vi "Generic command handler.vi"(8 "error in (no error)":errorcluster, 10 "Message in":refnum<class "GenericMessage.lvclass">, 11 "Cascade in":refnum<class "Cascade.lvclass">) -> (0 "error out":errorcluster, 2 "value":string, 3 "Cascade out":refnum<class "Cascade.lvclass">)   [LabVIEW 2012, in "Cascade.lvclass"]
doc: "The generic_command_handler processes the command 'generic'. Commands which are not part of the predefined list of commands fall under the 'generic' command for special activity."
uses:
  Cascade.lvclass
  <vilib>/Distrio/Murmex/GenericMessage/GenericMessage.lvclass
  <vilib>/Distrio/Murmex/Murmex/Murmex.lvclass
  Cascade.lvclass/Cascade.ctl
  <vilib>/Distrio/Murmex/ProceedMessage/ProceedMessage.lvclass
panel:
  # "This method is called when the GENERIC\ntrigger is sent. \n\nOverride this method when your component needs to\nrespond to this trigger. \n\nCall parent for proper implementation"
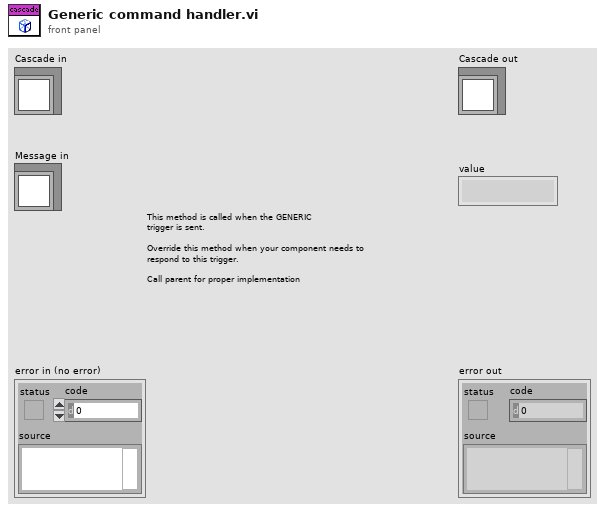
[diagram p1: front panel]
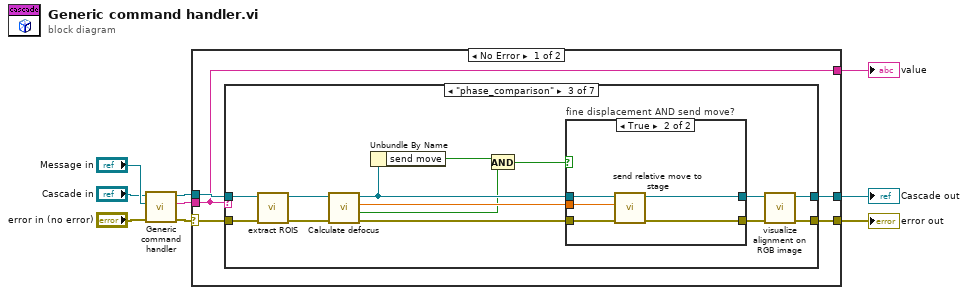
[diagram p0: block diagram]
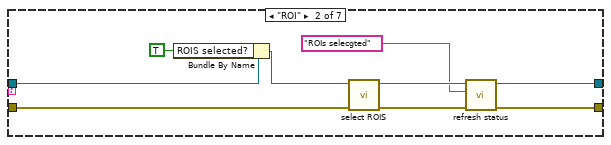
[diagram p3: hidden frame]
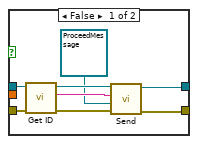
[diagram p4: hidden frame]
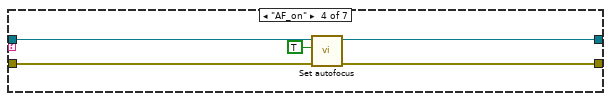
[diagram p5: hidden frame]
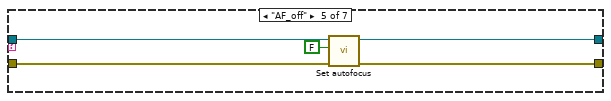
[diagram p6: hidden frame]
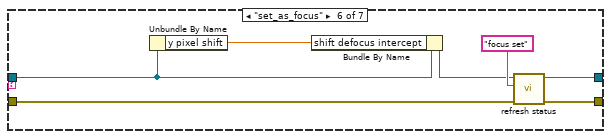
[diagram p7: hidden frame]
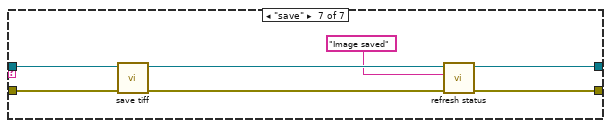
[diagram p8: hidden frame]
diagram:
  n1 = call-parent "Generic command handler.vi"("error in (no error)"="error in (no error)", "Message in"="Message in", "Murmex in"="Cascade in") -> ("error out"=w6:errorcluster, "value"=w4:string, "Murmex out"=w5:refnum<class "Cascade.lvclass">)  [unwired: 6 in]
  n2 = case shown="No Error" w6 {
    selector: w6 -> [w14 w78]
    tunnel: w5 -> [w13 w79]
    tunnel: w4 -> [w12 w77]
    tunnel: [w12 w77] -> w3
    tunnel: [w11 w78] -> w2
    tunnel: [w10 w79] -> w1
    frame No Error {
      n3 = case shown="\"phase_comparison\"" w12 {
        tunnel: w14 -> [w16 w23 w39 w57 w62 w64 w76]
        tunnel: w13 -> [w15 w19 w38 w55 w60 w66 w75]
        tunnel: [w16 w24 w29 w56 w61 w69 w73] -> w11
        tunnel: [w15 w25 w27 w54 w59 w68 w71] -> w10
        frame "False", Default {
        }
        frame "ROI" {
          n4 = Bundle By Name(cluster=w19, "ROIS selected?"=TRUE ("runtime.ROIS selected?")) -> (w18:refnum<class "Cascade.lvclass">)
          n5 = call-dynamic "select ROIS.vi"("error in (no error)"=w23, "Cascade in"=w18) -> ("error out"=w22:errorcluster, "Cascade out"=w21:refnum<class "Cascade.lvclass">)  [unwired: 8 in]
          n6 = call-dynamic "refresh status.vi"("error in (no error)"=w22, "String In"="ROIs selecgted", "Cascade in"=w21) -> ("error out"=w24:errorcluster, "Cascade out"=w25:refnum<class "Cascade.lvclass">)  [unwired: 7 in]
        }
        frame "phase_comparison" {
          n7 = call-dynamic "extract ROIS.vi"("error in (no error)"=w39, "Cascade in"=w38) -> ("error out"=w37:errorcluster, "Cascade out"=w35:refnum<class "Cascade.lvclass">)  [unwired: 8 in]
          n8 = call-dynamic "Calculate defocus.vi"("error in (no error)"=w37, "Cascade in"=w35) -> ("error out"=w36:errorcluster, "fine?"=w30:bool, "translation out"=w33:dbl[unit], "Cascade out"=w34:refnum<class "Cascade.lvclass">)  [unwired: 6 in]
          n9 = Unbundle By Name(w34) -> ("send move"=w32:bool)
          n10 = And(x=w32, y=w30) -> (x .and. y?=w31:bool)
          n11 = case "fine displacement AND send move?" shown="True" w31 {
            tunnel: [w44 w52] -> w28
            tunnel: [w45 w51] -> w26
            tunnel: w34 -> [w46 w50]
            tunnel: w36 -> [w47 w49]
            tunnel: w33 -> [_ w48]
            frame False {
              n12 = call <vilib>:"Get ID.vi"("error in (no error)"=w47, "Murmex in"=w46) -> ("error out"=w43:errorcluster, "component id"=w41:string, "Murmex out"=w42:refnum<class "Cascade.lvclass">)  [unwired: 7 in]
              n13 = call <vilib>:"Send.vi"("error in (no error)"=w43, "Message"=refnum<class "ProceedMessage.lvclass"> refnum ("Distrio Murmex 1.5:ProceedMessage"), "recipient"=w41, "Murmex in"=w42) -> ("error out"=w44:errorcluster, "Murmex out"=w45:refnum<class "Cascade.lvclass">)  [unwired: 6 in]
            }
            frame True {
              n14 = call-dynamic "send relative move to stage.vi"("error in (no error)"=w49, "move to send"=w48, "Cascade in"=w50) -> ("error out"=w52:errorcluster, "Cascade out"=w51:refnum<class "Cascade.lvclass">)  [unwired: 7 in]
            }
          }
          n15 = call-dynamic "visualize alignment on RGB image.vi"("error in (no error)"=w28, "Cascade in"=w26) -> ("error out"=w29:errorcluster, "Cascade out"=w27:refnum<class "Cascade.lvclass">)  [unwired: 8 in]
        }
        frame "AF_on" {
          n16 = call-dynamic "Set autofocus.vi"("error in (no error)"=w57, "autofocusing?"=TRUE, "Cascade in"=w55) -> ("error out"=w56:errorcluster, "Cascade out"=w54:refnum<class "Cascade.lvclass">)  [unwired: 7 in]
        }
        frame "AF_off" {
          n17 = call-dynamic "Set autofocus.vi"("error in (no error)"=w62, "autofocusing?"=FALSE, "Cascade in"=w60) -> ("error out"=w61:errorcluster, "Cascade out"=w59:refnum<class "Cascade.lvclass">)  [unwired: 7 in]
        }
        frame "set_as_focus" {
          n18 = Unbundle By Name(w66) -> ("y pixel shift"=w63:dbl)
          n19 = Bundle By Name(cluster=w66, "shift defocus intercept"=w63) -> (w65:refnum<class "Cascade.lvclass">)
          n20 = call-dynamic "refresh status.vi"("error in (no error)"=w64, "String In"="focus set", "Cascade in"=w65) -> ("error out"=w69:errorcluster, "Cascade out"=w68:refnum<class "Cascade.lvclass">)  [unwired: 7 in]
        }
        frame "save" {
          n21 = call-dynamic "save tiff.vi"("error in (no error)"=w76, "Cascade in"=w75) -> ("error out"=w74:errorcluster, "Cascade out"=w72:refnum<class "Cascade.lvclass">)  [unwired: 8 in]
          n22 = call-dynamic "refresh status.vi"("error in (no error)"=w74, "String In"="Image saved", "Cascade in"=w72) -> ("error out"=w73:errorcluster, "Cascade out"=w71:refnum<class "Cascade.lvclass">)  [unwired: 7 in]
        }
      }
    }
    frame Error {
    }
  }
  "error out" <- w2
  "Cascade out" <- w1
  "value" <- w3
